vi "trplot2.vi"(8 "Error In":errorcluster, 11 "T":dbl[][](array[numeric])=[[-0.4161468365471424, 0.9092974268256817, 3.0], [-0.9092974268256817, -0.4161468365471424, 1.0], [0.0, 0.0, 1.0]]) -> (0 "Error Out":errorcluster, 3 "XY Graph 2":cluster{dbl[], dbl[]}[](graph))   [LabVIEW 2013]
doc: "Given a 3x3 homogenous transformation (T) this function outputs a cluster of the plot components (TrPlot) needed to represent the transformation on an XY Graph."
uses:
  <vilib>/Analysis/coordinate.llb/2D Cartesian Coordinate Rotation (Scalar).vi
  <vilib>/Analysis/NI_AALPro.lvlib
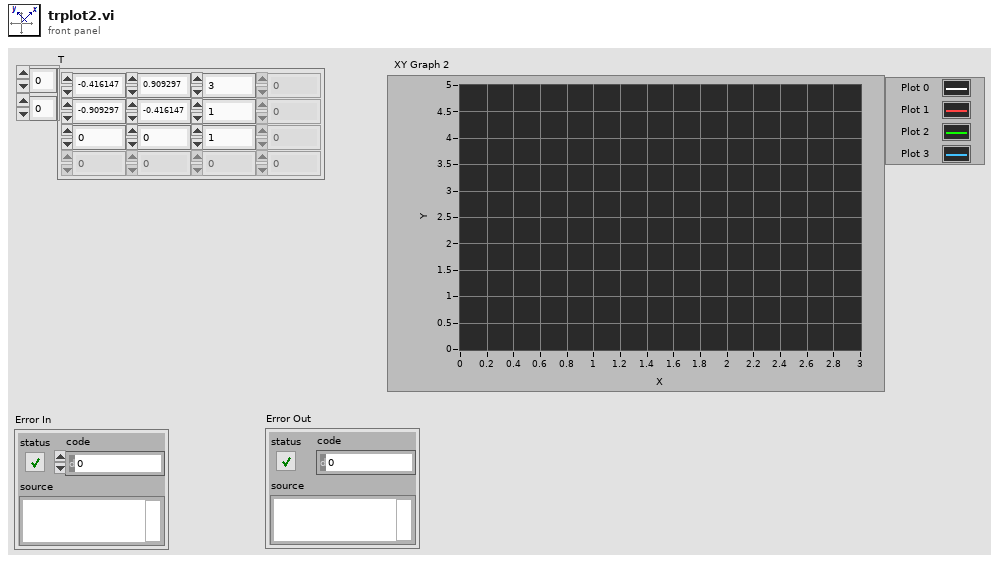
[diagram p1: front panel]
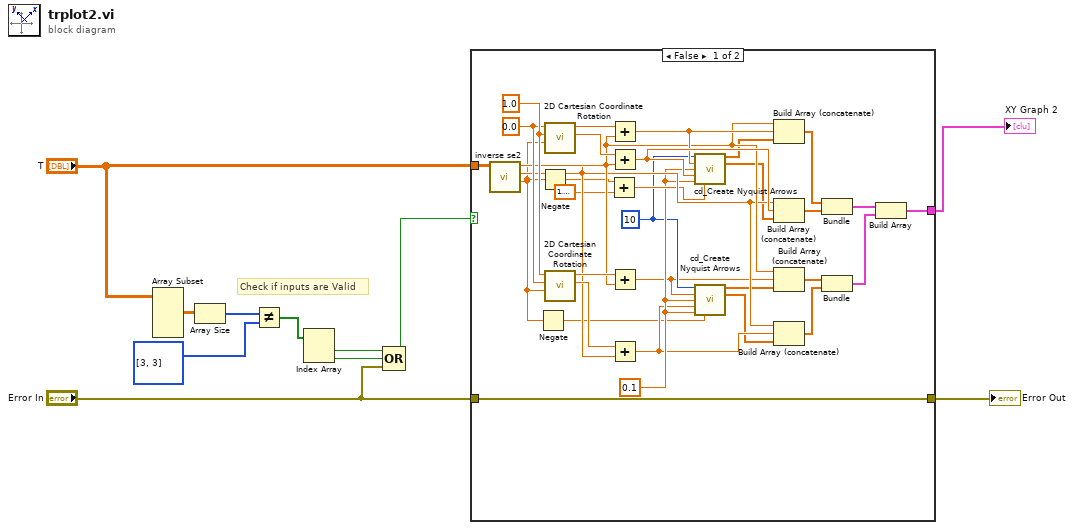
[diagram p0: block diagram]
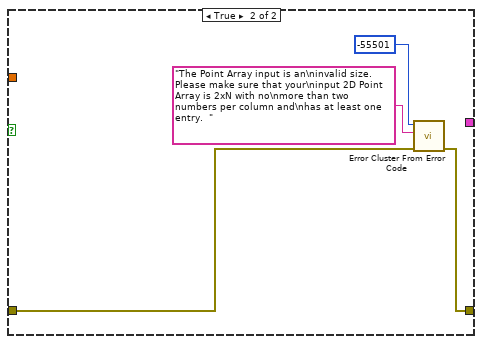
[diagram p2: hidden frame]
diagram:
  # "Check if inputs are Valid"
  n1 = Array Subset(array="T") -> (w11:dbl[][])  [unwired: 4 in]
  n2 = Array Size(array=w11) -> (size(s)=w9:i32[])
  n3 = Not Equal?(x=w9, y=i32[] [3, 3]) -> (x != y?=w7:bool[])
  n4 = Index Array(array=w7) -> (element #1=w6:bool, element #2=w5:bool)  [unwired: 2 in]
  n5 = Compound Arithmetic op=OR(w6, w5, "Error In") -> (w4:bool)
  n6 = case shown="False" w4 {
    tunnel: "T" -> [w37 _]
    tunnel: [w38 _] -> w1
    tunnel: "Error In" -> [w39 w45]
    tunnel: [w39 w44] -> w2
    frame False {
      w28 = 0.0 ("element")
      w29 = 1.0 ("element")
      w21 = 0.1 ("dx")
      w20 = 10 ("number of arrows")
      n7 = call "inverse se2.vi"("T"=w37) -> ("theta"=w18:dbl, "y"=w25:dbl, "x"=w26:dbl)  [unwired: 7 in, 1 out]
      n8 = Negate(x=w18) -> (-x=w12:dbl)
      n9 = Negate(x=w18) -> (-x=w13:dbl)
      n10 = call-poly <vilib>:"2D Cartesian Coordinate Rotation.vi"("theta"=w18, "y"=w29, "x"=w28) -> ("y out"=w30:dbl, "x out"=w34:dbl)  [unwired: 6 in, 1 out]
      n11 = call-poly <vilib>:"2D Cartesian Coordinate Rotation.vi"("theta"=w18, "y"=w28, "x"=w29) -> ("y out"=w35:dbl, "x out"=w36:dbl)  [unwired: 6 in, 1 out]
      n12 = Add(x=w13, y=1.5707963267948966) -> (x+y=w24:dbl)
      n13 = Add(x=w34, y=w26) -> (x+y=w27:dbl)
      n14 = Add(x=w30, y=w25) -> (x+y=w31:dbl)
      n15 = Add(x=w36, y=w26) -> (x+y=w19:dbl)
      n16 = Add(x=w35, y=w25) -> (x+y=w17:dbl)
      n17 = call <vilib>:"cd_Create Nyquist Arrows.vi"("number of arrows"=w20, "xo"=w27, "dx"=w21, "yo"=w31, "dy"=w21, "theta"=w24) -> ("array of x"=w23:dbl[], "array of y"=w22:dbl[])  [unwired: 8 in]
      n18 = call <vilib>:"cd_Create Nyquist Arrows.vi"("number of arrows"=w20, "xo"=w19, "dx"=w21, "yo"=w17, "dy"=w21, "theta"=w12) -> ("array of x"=w15:dbl[], "array of y"=w14:dbl[])  [unwired: 8 in]
      n19 = Build Array (concatenate)(w26, w27, w23) -> (w43:dbl[])
      n20 = Build Array (concatenate)(w25, w31, w22) -> (w42:dbl[])
      n21 = Build Array (concatenate)(w26, w19, w15) -> (w40:dbl[])
      n22 = Build Array (concatenate)(w25, w17, w14) -> (w41:dbl[])
      n23 = Bundle(w43, w42) -> (w33:cluster{dbl[], dbl[]})  [unwired: 1 in]
      n24 = Bundle(w40, w41) -> (w32:cluster{dbl[], dbl[]})  [unwired: 1 in]
      n25 = Build Array(w33, w32) -> (w38:cluster{dbl[], dbl[]}[])
    }
    frame True {
      n26 = call <vilib>:"Error Cluster From Error Code.vi"("error in (no error)"=w45, "error message (\"\")"="The Point Array input is an\ninvalid size. Please make sure that your\ninput 2D Point Array is 2xN with no\nmore than two numbers per column and\nhas at least one entry.  " ("error message (\"\")"), "error code (0)"=-55501) -> ("error out"=w44:errorcluster)  [unwired: 6 in]
    }
  }
  "Error Out" <- w2
  "XY Graph 2" <- w1
